vi "Bump_Counter.vi"(0 "ref":dbl, 2 "D-Pad":i16, 3 "quanta":dbl, 4 "reset":bool) -> (5 "out":dbl)   [LabVIEW 2016]
doc: "Description:\nThis subVI provides discrete stepped control of an output value relative to an initial reference value. The output is quantized at a user specified level.\n\nInputs:\nREF - Reference value, and initial value of OUT prior to adding bump values.\nRESET - Erases the bumps on the rising edge and returns OUT to the value REF, suspending further bumping while it is True.\nThe bumping function resumes when RESET becomes False.\nCNTRL - Control input value which is monitored for transition point crossings. Crossing from the dead-band to over the +0.5 point \nwill increase OUT by one QUANTA. Transitioning over the -0.5 point decreases OUT by one QUANTA.\nQUANTA - The discrete step value used to change OUT each time CNTRL crosses a transition point. Provides a designed level of precision for commanded changes to OUT.\n\nOutputs:\nOUT - Reference value modified by commanded count of quantum bumps."
uses:
  <vilib>/Rock Robotics/WPI/Joystick/WPI_JoystickDeviceEnum.ctl
  <vilib>/Rock Robotics/WPI/Joystick/WPI_JoystickAxis.ctl
panel:
  out "Out":dbl
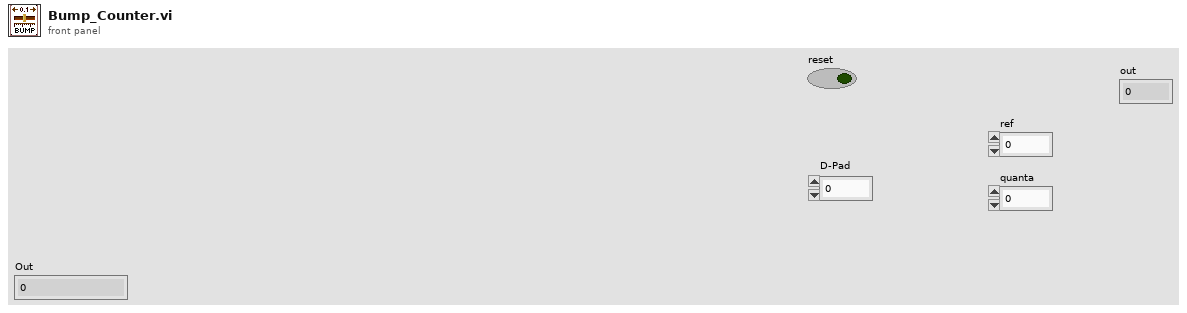
[diagram p1: front panel]
types:
  T1 = typedef "WPI_JoystickAxis.ctl" = enum16{"Axis 0", "Axis 1", "Axis 2", "Axis 3", "Axis 4", "Axis 5"}
  T2 = typedef "WPI_JoystickDevRef.ctl" = cluster{"Device":T3}
  T3 = typedef "WPI_JoystickDeviceEnum.ctl" = enum16{"USB 0", "USB 1", "USB 2", "USB 3", "USB 4", "USB 5"}
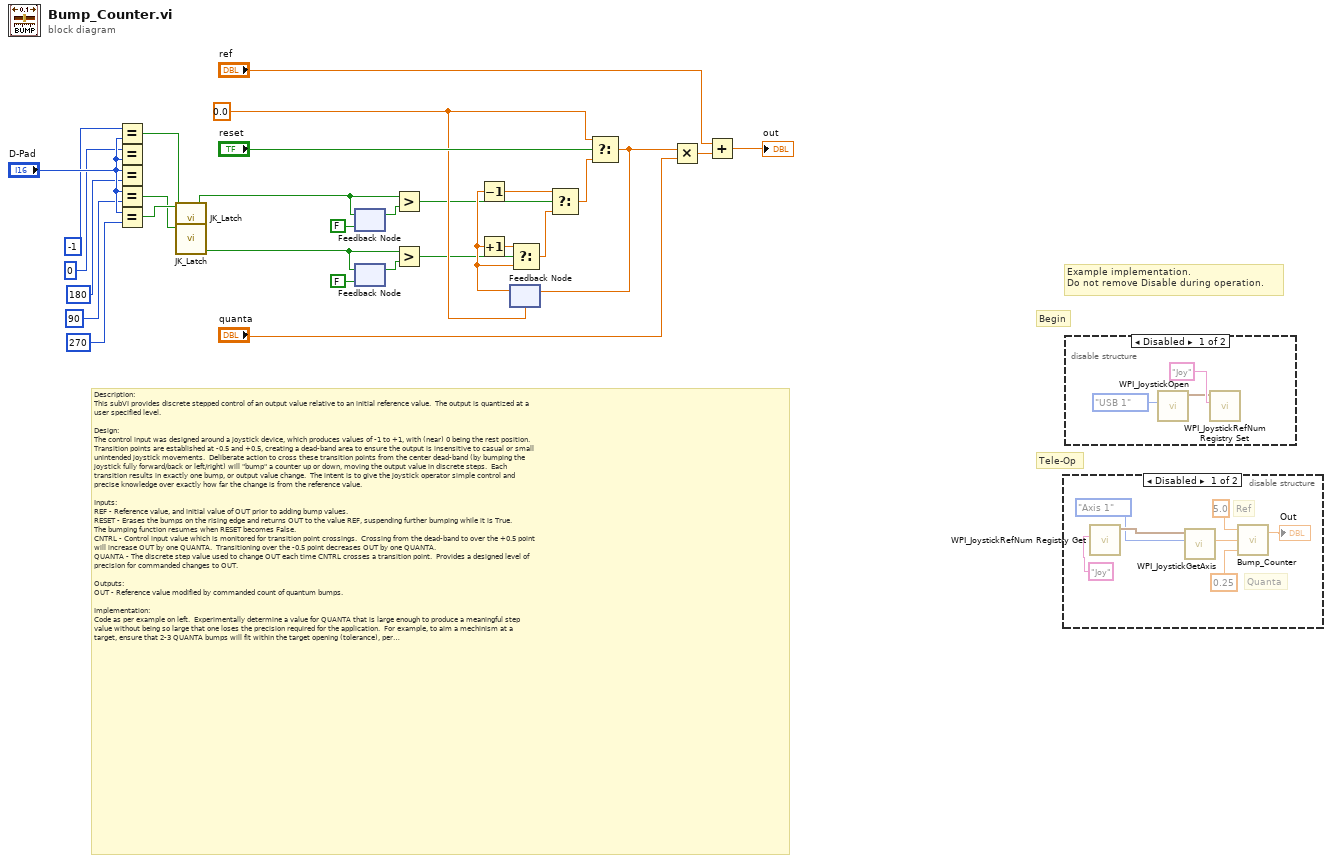
[diagram p0: block diagram]
diagram:
  w15 = 0.0 ("initial")
  # "Begin"
  # "Tele-Op"
  # "Example implementation.\nDo not remove Disable during operation."
  # "Description:\nThis subVI provides discrete stepped control of an output value relative to an initial reference value.  The output is quantized at a \nuser specified level.\n\nDesign:\nThe control input was designed around a joystick device, which produces values of -1 to +1, with (near) 0 being the rest position.  \nTransition points are established at -0.5 and +0.5, creating a dead-band area to ensure the output is insensitive to casual or small\nunintended joystick movements.  Deliberate action to cross these transition points from the center dead-band (by bumping the\njoystick fully forward/back or left/right) will \"bump\" a counter up or down, moving the output value in discrete steps.  Each \ntransition results in exactly one bump, or output value change.  The intent is to give the joystick operator simple control and \nprecise knowledge over exactly how far the change is from the reference value.\n\nInputs:\nREF - Reference value, and initial value of OUT prior to adding bump values.\nRESET - Erases the bumps on the rising edge and returns OUT to the value REF, suspending further bumping while it is True.\nThe bumping function resumes when RESET becomes False.\nCNTRL - Control input value which is monitored for transition point crossings.  Crossing from the dead-band to over the +0.5 point \nwill increase OUT by one QUANTA.  Transitioning over the -0.5 point decreases OUT by one QUANTA.\nQUANTA - The discrete step value used to change OUT each time CNTRL crosses a transition point.  Provides a designed level of\nprecision for commanded changes to OUT.\n\nOutputs:\nOUT - Reference value modified by commanded count of quantum bumps. \n\nImplementation:\nCode as per example on left.  Experimentally determine a value for QUANTA that is large enough to produce a meaningful step \nvalue without being so large that one loses the precision required for the application.  For example, to aim a mechinism at a \ntarget, ensure that 2-3 QUANTA bumps will fit within the target opening (tolerance), perhaps at low, mid, and high positions \nwithin the opening ... however, don't make QUANTA so small that it takes 'all day' to make an adjustment!\n\n----- RoboBees Team 836! -----  You too can change things ... consider a career in STEM!"
  n1 = Equal?(x=i64 -1, y="D-Pad") -> (x = y?=w4:bool)
  n2 = Equal?(x=i64 0, y="D-Pad") -> ()  [unwired: 1 out]
  n3 = Equal?(x="D-Pad", y=i64 180) -> ()  [unwired: 1 out]
  n4 = Equal?(x="D-Pad", y=i64 90) -> (x = y?=w1:bool)
  n5 = Equal?(x="D-Pad", y=i64 270) -> (x = y?=w5:bool)
  n6 = call <userlib>:"JK_Latch.vi"("Reset"=w4, "Set"=w5) -> ("Q"=w3:bool)  [unwired: 5 in]
  n7 = call <userlib>:"JK_Latch.vi"("Reset"=w4, "Set"=w1) -> ("Q"=w2:bool)  [unwired: 5 in]
  n8 = feedback #1(FALSE ("down")) -> (w26:bool)
  n9 = feedback-in #1(w3) -> ()
  n10 = feedback #2(FALSE ("down")) -> (w23:bool)
  n11 = feedback-in #2(w2) -> ()
  n12 = Greater?(x=w3, y=w26) -> (0:w13:bool)
  n13 = Greater?(x=w2, y=w23) -> (0:w12:bool)
  n14 = feedback #3(w15) -> (w21:dbl)
  n15 = Decrement(x=w21) -> (x-1=w28:dbl)
  n16 = Increment(x=w21) -> (x+1=w27:dbl)
  n17 = Select(t=w27, s=w12, f=w21) -> (s? t:f=w29:dbl)
  n18 = Select(t=w28, s=w13, f=w29) -> (s? t:f=w20:dbl)
  n19 = Select(t=w15, s="reset", f=w20) -> (s? t:f=w14:dbl)
  n20 = feedback-in #3(w14) -> ()
  n21 = Multiply(x=w14, y="quanta") -> (x*y=w18:dbl)
  n22 = Add(x="ref", y=w18) -> (x+y=→"out":dbl)
  n23 = disable-structure shown="Disabled" {
    frame Disabled {
      # "Ref"
      # "Quanta"
      n24 = call <vilib>:"WPI_JoystickRefNum Registry Get.vi"("refnum name"="Joy") -> ("JoystickDevRef"=w34:T2)  [unwired: 9 in, 1 out]
      n25 = call <vilib>:"WPI_JoystickGetAxis.vi"("Axis"=WPI_JoystickAxis."Axis 1", "JoystickDevRef"=w34) -> ("Value"=w32:dbl)  [unwired: 8 in, 1 out]
      n26 = call "Bump_Counter.vi"("ref"=5.0, "D-Pad"=w32, "quanta"=0.25) -> ("out"=→"Out":dbl)  [unwired: 3 in]
    }
    frame Enabled {
    }
  }
  n27 = disable-structure shown="Disabled" {
    frame Disabled {
      n28 = call <vilib>:"WPI_JoystickOpen.vi"("JoystickDevice"=WPI_JoystickDeviceEnum."USB 1") -> ("JoystickDevRef"=w38:T2)  [unwired: 10 in]
      n29 = call <vilib>:"WPI_JoystickRefNum Registry Set.vi"("refnum name"="Joy", "JoystickDevRef"=w38) -> ()  [unwired: 8 in, 2 out]
    }
    frame Enabled {
    }
  }
